vi "Close_connection.vi"(8 "error in (no error)":errorcluster, 11 "DB_SQLite in":refnum<class "DB_SQLite.lvclass">) -> (0 "error out":errorcluster, 3 "DB_SQLite out":refnum<class "DB_SQLite.lvclass">)   [LabVIEW 2015, in "DB_SQLite.lvclass"]
uses:
  DB_SQLite.lvclass
  <vilib>/drjdpowell/SQLite Library/SQL Connection/Connection.lvclass
  DB.lvclass
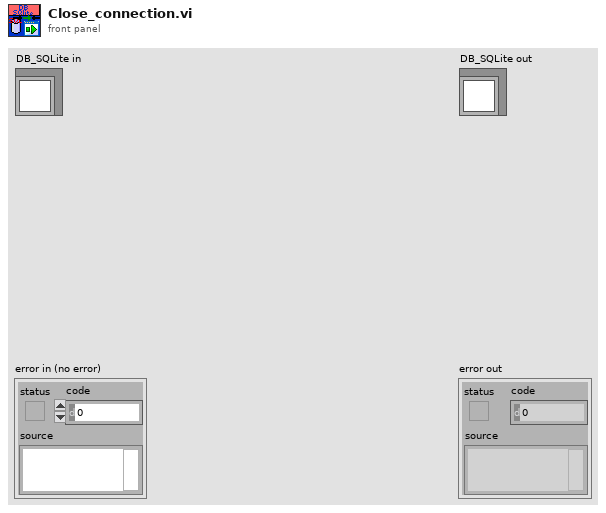
[diagram p1: front panel]
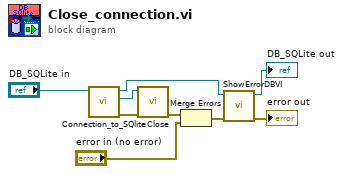
[diagram p0: block diagram]
diagram:
  n1 = call "Connection_to_SQlite.vi"("DB_SQLite in"="DB_SQLite in") -> ("error out"=w8:errorcluster, "SQlite connection"=w7:refnum<class "Connection.lvclass">, "DB_SQLite out"=w3:refnum<class "DB_SQLite.lvclass">)  [unwired: 8 in]
  n2 = call-dynamic "Close.vi"("error in (no error)"=w8, "SQLite Connection in"=w7) -> ("error out"=w6:errorcluster)  [unwired: 9 in]
  n3 = Merge Errors(w6, "error in (no error)") -> (w4:errorcluster)
  n4 = call "ShowErrorDBVI.vi"("error in (no error)"=w4, "DB in"=w3) -> ("error out"=→"error out":errorcluster, "DB out"=→"DB_SQLite out":refnum<class "DB_SQLite.lvclass">)  [unwired: 8 in]
